vi "SSS_V1.0(TEST).vi"() -> ()   [LabVIEW 2017]
uses:
  <vilib>/DAQmx/configure/timing.llb/DAQmx Timing (Sample Clock).vi
  <vilib>/Analysis/NI_AALBase.lvlib
  <vilib>/Analysis/3filter.llb/FIR Filter (DBL).vi
  <vilib>/DAQmx/read.llb/DAQmx Read (Analog 1D Wfm NChan NSamp).vi
  <vilib>/DAQmx/write.llb/DAQmx Write (Analog Wfm 1Chan NSamp).vi
  <vilib>/measure/NI_MAPro.lvlib
  <vilib>/measure/maspectr.llb/FFT Power Spectrum and PSD for 1 Chan.vi
  <vilib>/measure/maspectr.llb/Power Spectrum and PSD Export Mode.ctl
  <vilib>/DAQmx/create/channels.llb/DAQmx Create Channel (AI-Voltage-Basic).vi
  <vilib>/DAQmx/create/channels.llb/DAQmx Create Channel (AO-Voltage-Basic).vi
panel:
  out "TX Spectrum":cluster{"f0":dbl, "df":dbl, "magnitude":dbl[]}(graph)
  out "TX Signal":waveform(dbl)(graph)
  out "RX Result 2":waveform(dbl)(graph)
  out "Signal Processing Result":waveform(dbl)(graph)
  in  "송신 채널 설정":tag="Dev3/ao0"
  in  "송신 디바이스 이름":tag="Dev3"
  in  "Pulse length(sec)":dbl=0.0004 format="%#_6p"
  in  "Stop Frequency(Hz)":dbl=470000.0 format="%#_6p"
  in  "Start Frequency(Hz)":dbl=430000.0 format="%#_6p"
  in  "Number of Sample":i32=150000
  out "RX.CH2":waveform(dbl)(graph)
  out "RX.CH1":waveform(dbl)(graph)
  in  "RX Time(sec)":dbl=2.0
  in  "수신 디바이스 이름":tag="Dev3"
  in  "수신 채널 설정":tag="Dev3/ai0:1"
  in  "sampling rate":dbl=1500000.0 caption="Sampling Frequency" format="%0.2f"
  in  "sample mode":i32(ring)=10123 caption="샘플 모드" items=["유한 샘플"=10178, "연속 샘플"=10123, "하드웨어 타이밍에 의한 단일 포인트"=12522]
  # "TX Variable Setting"
  # "ADC/DAC Setting"
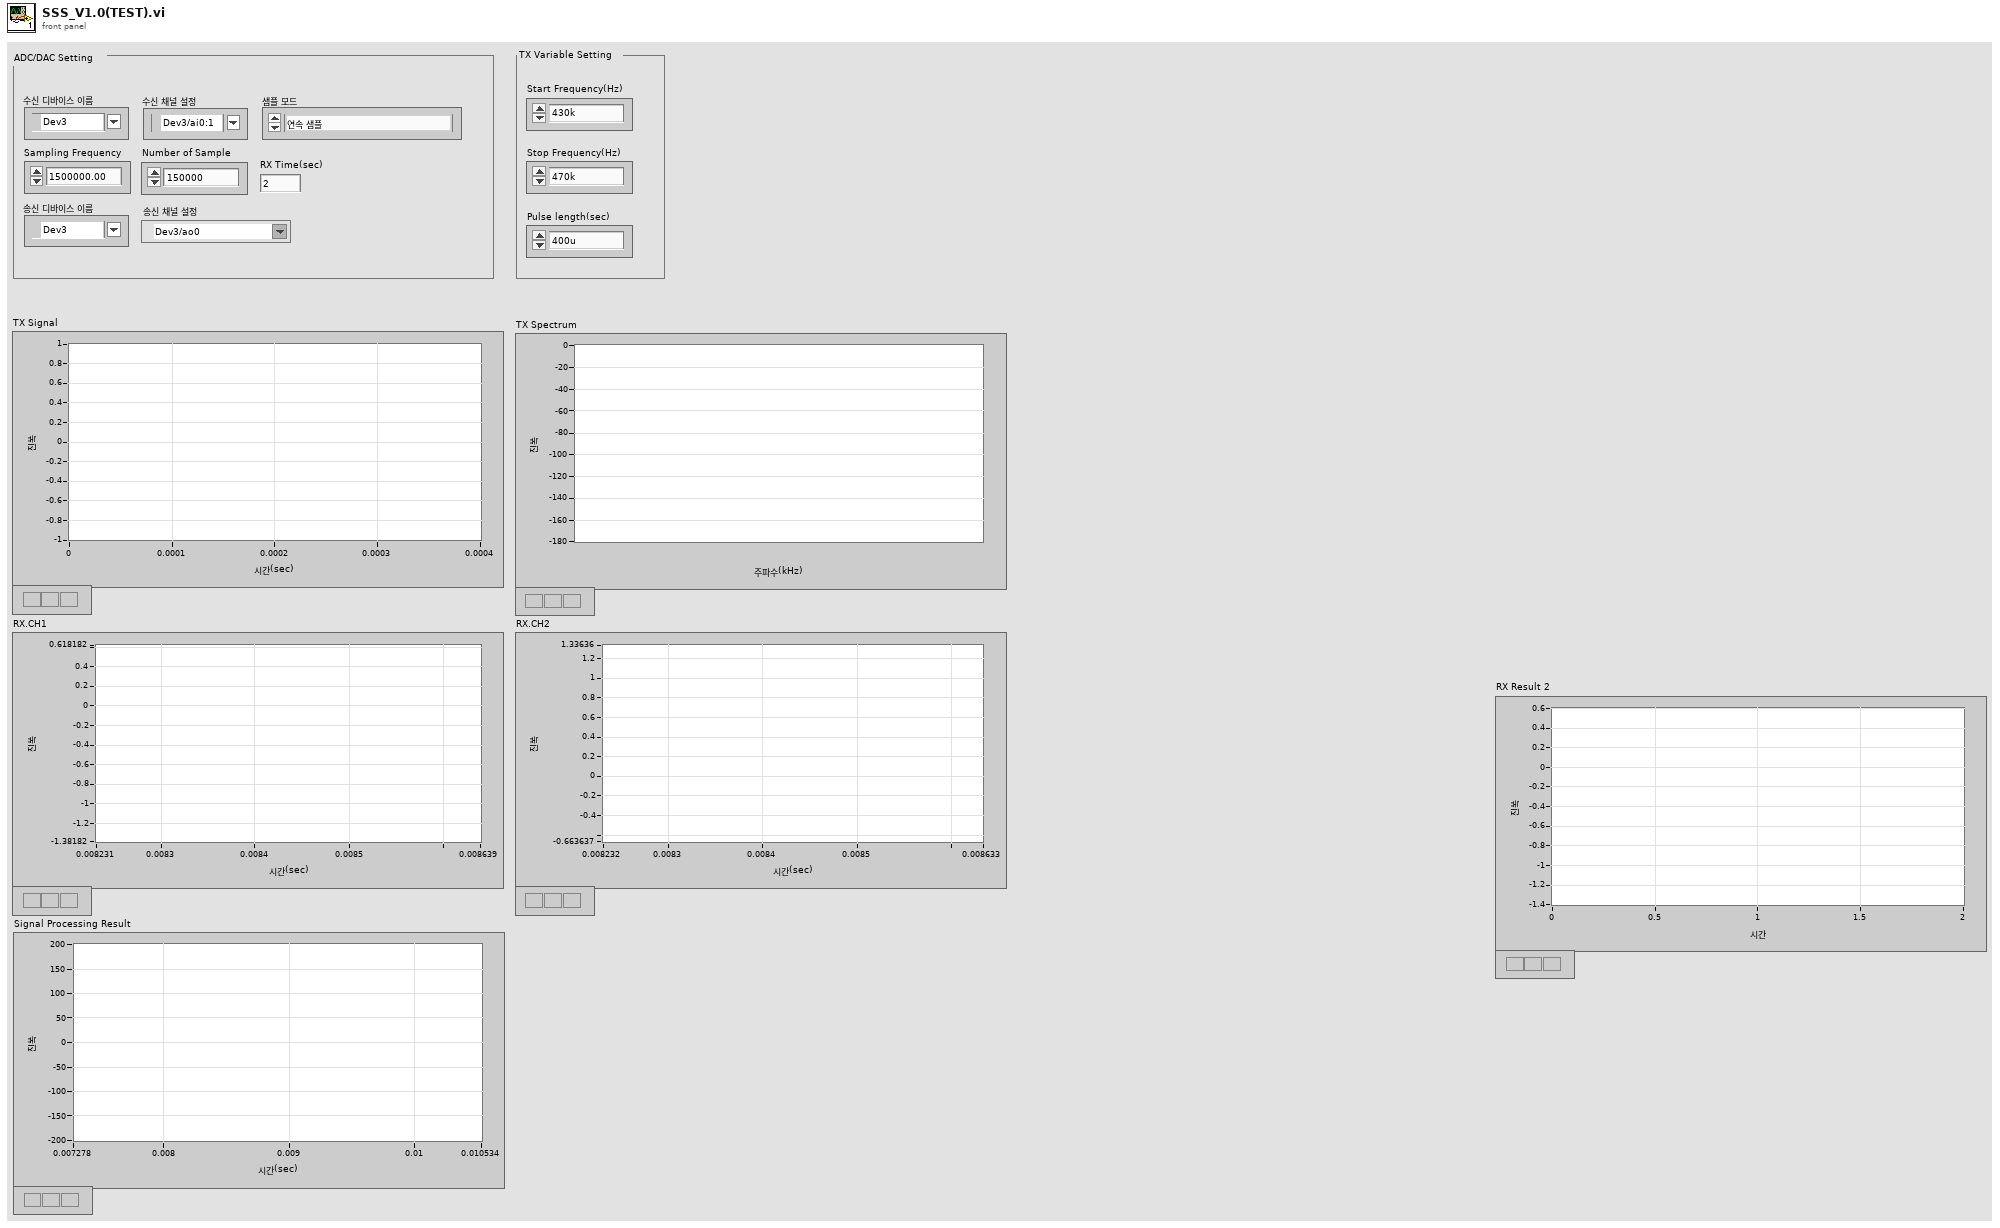
[diagram p1: front panel]
types:
  T1 = typedef "NI_MAPro.lvlib/Power Spectrum and PSD Export Mode.ctl" = u16
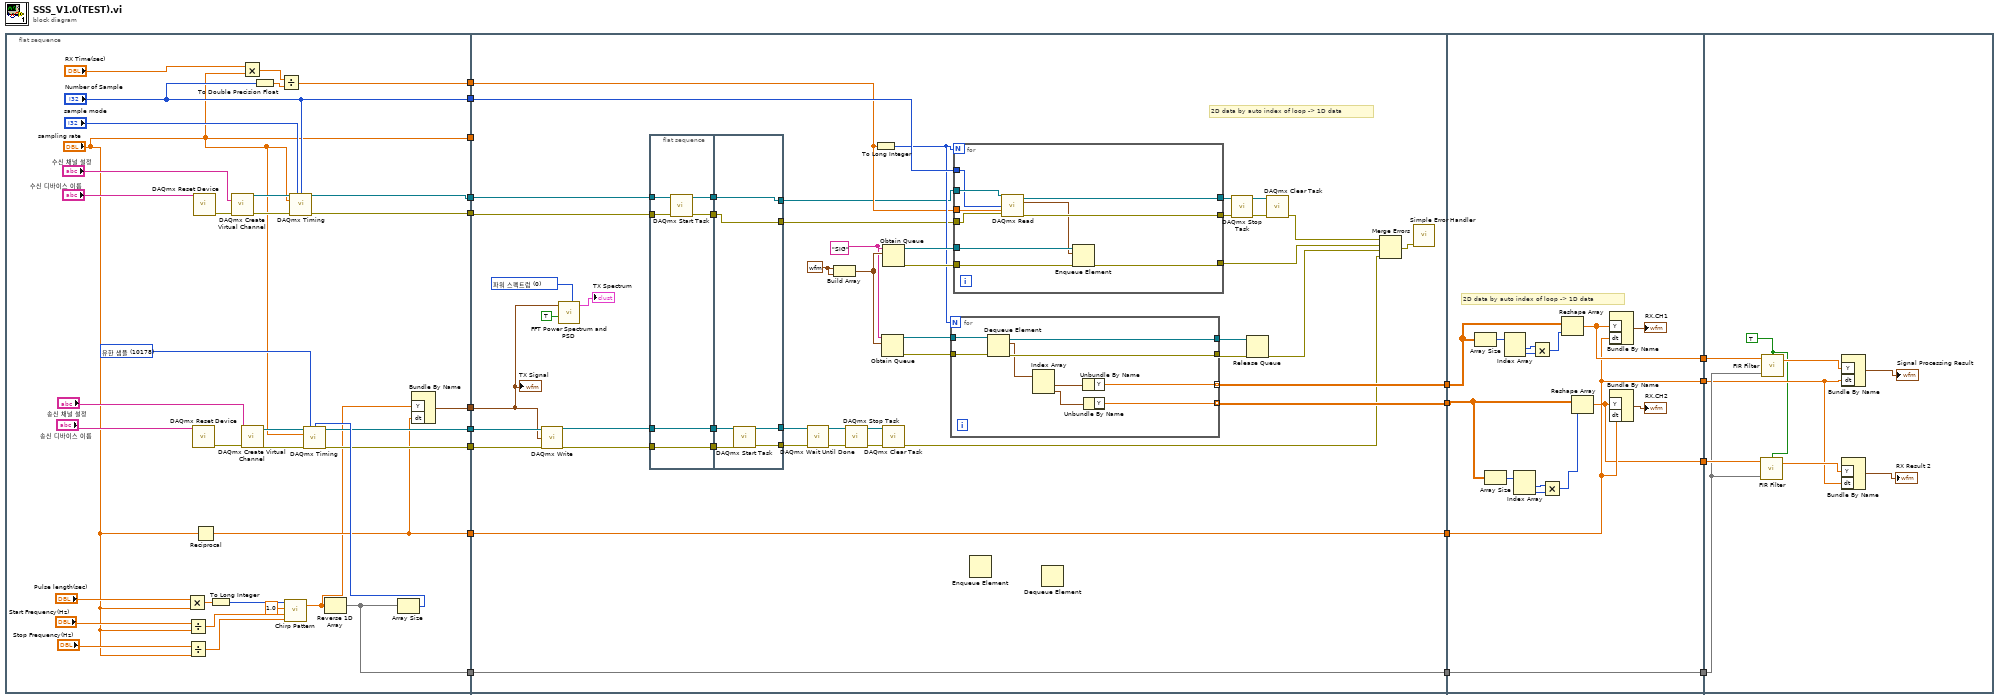
[diagram p0: block diagram]
diagram:
  n1 = flat-sequence {
    tunnel: ["sampling rate"] -> w18
    tunnel: ["Number of Sample"] -> w17
    tunnel: [w43] -> w16
    tunnel: [w42] -> w15
    tunnel: [w41] -> w14
    tunnel: [w23] -> w11
    tunnel: [w26] -> w9
    tunnel: [w25] -> w8
    tunnel: [w22] -> w7
    tunnel: [w20] -> w5
    tunnel: w18 -> [_]
    tunnel: w17 -> [w87]
    tunnel: w16 -> [w73]
    tunnel: w15 -> [w78]
    tunnel: w14 -> [w85]
    tunnel: [w80] -> w13
    tunnel: [w79] -> w12
    tunnel: w11 -> [w54]
    tunnel: [w54] -> w10
    tunnel: w9 -> [w72]
    tunnel: w8 -> [w71]
    tunnel: w7 -> [w58]
    tunnel: w5 -> [w59]
    tunnel: [w59] -> w4
    tunnel: w13 -> [w143]
    tunnel: w12 -> [w138]
    tunnel: w10 -> [w134]
    tunnel: [w136] -> w6
    tunnel: w4 -> [w135]
    tunnel: [w135] -> w3
    tunnel: [w134] -> w2
    tunnel: [w133] -> w1
    tunnel: w6 -> [w156]
    tunnel: w3 -> [w150]
    tunnel: w2 -> [w149]
    tunnel: w1 -> [w151]
    frame #0 {
      w29 = 10178 items=["유한 샘플"=10178, "연속 샘플"=10123, "하드웨어 타이밍에 의한 단일 포인트"=12522] ("sample mode")
      n2 = Multiply(x="Pulse length(sec)", y="sampling rate") -> (x*y=w39:dbl)
      n3 = Divide(x="Start Frequency(Hz)", y="sampling rate") -> (x/y=w36:dbl)
      n4 = Divide(x="Stop Frequency(Hz)", y="sampling rate") -> (x/y=w33:dbl)
      n5 = call <vilib>:"DAQmx Reset Device.vi"("device in"="송신 디바이스 이름") -> ("error out"=w32:errorcluster)  [unwired: 1 in, 13 out]
      n6 = call <vilib>:"DAQmx Reset Device.vi"("device in"="수신 디바이스 이름") -> ("error out"=w47:errorcluster)  [unwired: 1 in, 13 out]
      n7 = Reciprocal(x="sampling rate") -> (1/x=w23:dbl)
      n8 = To Long Integer(number=w39) -> (32bit integer=w38:i32)
      n9 = call-poly <vilib>:"DAQmx Create Virtual Channel.vi"("physical channels"="수신 채널 설정", "error in"=w47) -> ("task out"=w46:refnum<k21>, "error out"=w45:errorcluster)  [unwired: 7 in, 5 out]
      n10 = Multiply(x="RX Time(sec)", y="sampling rate") -> (x*y=w50:dbl)
      n11 = call-poly <vilib>:"DAQmx Create Virtual Channel.vi"("physical channels"="송신 채널 설정", "error in"=w32) -> ("task out"=w28:refnum<k21>, "error out"=w31:errorcluster)  [unwired: 7 in, 5 out]
      n12 = To Double Precision Float(number="Number of Sample") -> (double precision float=w51:dbl)
      n13 = Divide(x=w50, y=w51) -> (x/y=w41:dbl)
      n14 = call <vilib>:"Chirp Pattern.vi"("f2"=w33, "f1"=w36, "amplitude"=1.0, "samples"=w38) -> ("Chirp Pattern"=w19:dbl[])  [unwired: 1 out]
      n15 = call-poly <vilib>:"DAQmx Timing.vi"("task/channels in"=w46, "sample mode"="sample mode", "samples per channel"="Number of Sample", "rate"="sampling rate", "error in"=w45) -> ("task out"=w43:refnum<k21>, "error out"=w42:errorcluster)  [unwired: 2 in, 7 out]
      n16 = Reverse 1D Array(array=w19) -> (reversed array=w20:dbl[])
      n17 = Array Size(array=w20) -> (size(s)=w30:i32)
      n18 = call-poly <vilib>:"DAQmx Timing.vi"("task/channels in"=w28, "sample mode"=w29, "samples per channel"=w30, "rate"="sampling rate", "error in"=w31) -> ("task out"=w26:refnum<k21>, "error out"=w25:errorcluster)  [unwired: 2 in, 7 out]
      n19 = Bundle By Name("Y"=w19, "dt"=w23) -> (w22:waveform(dbl))  [unwired: 1 in]
    }
    frame #1 {
      w56 = T1 0 items=["파워 스펙트럼", "파워 스펙트럼 밀도"] ("export mode")
      w84 = "SIG" ("이름(이름없음)")
      w89 = waveform(dbl) {"t0"=timestamp(0 s since 1904-01-01), "dt"=1.0, "Y"=[]} ("Waveform")
      # "2D data by auto index of loop -> 1D data"
      n20 = call-poly <vilib>:"DAQmx Write.vi"("task/channels in"=w72, "data"=w58, "error in"=w71) -> ("task out"=w68:refnum<k21>, "error out"=w70:errorcluster)  [unwired: 10 in, 1 out]
      n21 = call-poly <vilib>:"FFT Power Spectrum and PSD.vi"("export mode"=w56, "dB On (F)"=TRUE, "time signal"=w58) -> ("Power Spectrum / PSD"=→"TX Spectrum":cluster{"f0":dbl, "df":dbl, "magnitude":dbl[]})  [unwired: 5 in, 3 out]
      n22 = flat-sequence {
        tunnel: w78 -> [w106]
        tunnel: [w105] -> w77
        tunnel: [w104] -> w74
        tunnel: w73 -> [w103]
        tunnel: w70 -> [w102]
        tunnel: [w102] -> w69
        tunnel: w68 -> [w101]
        tunnel: [w101] -> w67
        tunnel: w77 -> [w112]
        tunnel: [w112] -> w76
        tunnel: [w111] -> w75
        tunnel: w74 -> [w111]
        tunnel: w69 -> [w110]
        tunnel: w67 -> [w109]
        tunnel: [w108] -> w62
        tunnel: [w107] -> w61
        frame #0 {
          n23 = call <vilib>:"DAQmx Start Task.vi"("task/channels in"=w103, "error in"=w106) -> ("task out"=w104:refnum<k21>, "error out"=w105:errorcluster)  [unwired: 12 in]
        }
        frame #1 {
          n24 = call <vilib>:"DAQmx Start Task.vi"("task/channels in"=w109, "error in"=w110) -> ("task out"=w108:refnum<k21>, "error out"=w107:errorcluster)  [unwired: 12 in]
        }
      }
      n25 = call <vilib>:"DAQmx Wait Until Done.vi"("task/channels in"=w62, "error in"=w61) -> ("task out"=w64:refnum<k21>, "error out"=w63:errorcluster)  [unwired: 12 in]
      n26 = Build Array(w89, w89) -> (w88:waveform(dbl)[])
      n27 = call <vilib>:"DAQmx Stop Task.vi"("task/channels in"=w64, "error in"=w63) -> ("task out"=w66:refnum<k21>, "error out"=w65:errorcluster)  [unwired: 12 in]
      n28 = To Long Integer(number=w85) -> (32bit integer=w86:i32)
      n29 = Obtain Queue(name (unnamed)=w84, element data type=w88) -> (queue out=w92:refnum<queue>, error out=w91:errorcluster)  [unwired: 3 in, 1 out]
      n30 = Obtain Queue(name (unnamed)=w84, element data type=w88) -> (queue out=w98:refnum<queue>, error out=w97:errorcluster)  [unwired: 3 in, 1 out]
      n31 = call <vilib>:"DAQmx Clear Task.vi"("task in"=w66, "error in"=w65) -> ("error out"=w60:errorcluster)  [unwired: 13 in]
      n32 = for {
        N: w86 -> [_]
        tunnel: w92 -> [w121]
        tunnel: w91 -> [w120]
        tunnel: [w119] -> w83
        tunnel: [w117] -> w81
        tunnel: [w114] -> w80 mode=indexing
        tunnel: [w115] -> w79 mode=indexing
        n33 = Dequeue Element(queue=w121, error in (no error)=w120) -> (queue out=w117:refnum<queue>, element=w118:waveform(dbl)[], error out=w119:errorcluster)  [unwired: 1 in, 1 out]
        n34 = Index Array(array=w118) -> (element #1=w116:waveform(dbl), element #2=w113:waveform(dbl))  [unwired: 2 in]
        n35 = Unbundle By Name(w116) -> ("Y"=w114:dbl[])
        n36 = Unbundle By Name(w113) -> ("Y"=w115:dbl[])
      }
      n37 = for {
        N: w86 -> [_]
        tunnel: w98 -> [w131]
        tunnel: w97 -> [w130]
        tunnel: [w129] -> w95
        tunnel: [w128] -> w94
        tunnel: [w127] -> w93
        tunnel: w75 -> [w125]
        tunnel: w76 -> [w124]
        tunnel: w87 -> [w123]
        tunnel: w85 -> [w122]
        n38 = call-poly <vilib>:"DAQmx Read.vi"("task/channels in"=w125, "number of samples per channel"=w123, "timeout"=w122, "error in"=w124) -> ("task out"=w128:refnum<k21>, "data"=w126:waveform(dbl)[], "error out"=w127:errorcluster)  [unwired: 9 out]
        n39 = Enqueue Element(queue=w131, element=w126, error in (no error)=w130) -> (error out=w129:errorcluster)  [unwired: 1 in, 2 out]
      }
      n40 = Enqueue Element() -> ()  [unwired: 4 in, 3 out]
      n41 = Dequeue Element() -> ()  [unwired: 3 in, 4 out]
      n42 = call <vilib>:"DAQmx Stop Task.vi"("task/channels in"=w94, "error in"=w93) -> ("task out"=w99:refnum<k21>, "error out"=w100:errorcluster)  [unwired: 12 out]
      n43 = Release Queue(queue=w81, error in (no error)=w83) -> (error out=w82:errorcluster)  [unwired: 3 out]
      n44 = call <vilib>:"DAQmx Clear Task.vi"("task in"=w99, "error in"=w100) -> ("error out"=w96:errorcluster)  [unwired: 13 out]
      n45 = Merge Errors(w96, w95, w82, w60) -> (w90:errorcluster)
      n46 = call <vilib>:"Simple Error Handler.vi"("error in (no error)"=w90) -> ()  [unwired: 4 in, 5 out]
      "TX Signal" <- w58
    }
    frame #2 {
      # "2D data by auto index of loop -> 1D data"
      n47 = Array Size(array=w143) -> (size(s)=w144:i32[])
      n48 = Array Size(array=w138) -> (size(s)=w139:i32[])
      n49 = Index Array(array=w144) -> (element #1=w146:i32, element #2=w145:i32)  [unwired: 2 in]
      n50 = Index Array(array=w139) -> (element #1=w141:i32, element #2=w140:i32)  [unwired: 2 in]
      n51 = Multiply(x=w146, y=w145) -> (x*y=w147:i32)
      n52 = Multiply(x=w141, y=w140) -> (x*y=w142:i32)
      n53 = Reshape Array(w143, w147) -> (w136:dbl[])
      n54 = Reshape Array(w138, w142) -> (w133:dbl[])
      n55 = Bundle By Name("Y"=w136, "dt"=w134) -> (→"RX.CH1":waveform(dbl))  [unwired: 1 in]
      n56 = Bundle By Name("Y"=w133, "dt"=w134) -> (→"RX.CH2":waveform(dbl))  [unwired: 1 in]
    }
    frame #3 {
      w148 = TRUE ("init/cont (init:F)")
      n57 = call-poly <vilib>:"FIR Filter.vi"("init/cont (init:F)"=w148, "FIR Coefficients"=w150, "X"=w151) -> ("Filtered X"=w153:dbl[])  [unwired: 1 in, 1 out]
      n58 = call-poly <vilib>:"FIR Filter.vi"("init/cont (init:F)"=w148, "FIR Coefficients"=w150, "X"=w156) -> ("Filtered X"=w155:dbl[])  [unwired: 1 in, 1 out]
      n59 = Bundle By Name("Y"=w153, "dt"=w149) -> (→"RX Result 2":waveform(dbl))  [unwired: 1 in]
      n60 = Bundle By Name("Y"=w155, "dt"=w149) -> (→"Signal Processing Result":waveform(dbl))  [unwired: 1 in]
    }
  }
